vi "UTILITY Array Get 1D Column From 2D.vi"(0 "2D Array Data":dbl[][](array[numeric])=[[4000.0, 0.760276], [4100.0, 0.729117], [4200.0, 0.722886], [4300.0, 0.729117], [4400.0, 0.735349], [4500.0, 0.735349], [4600.0, 0.735349], [4700.0, 0.835058], [4800.0, 0.841289], [4900.0, 0.928534], [5000.0, 0.947229], [5100.0, 1.015779], [5200.0, 1.065633], [5300.0, 1.140414], [5400.0, 1.333599], [5500.0, 1.302441], [5600.0, 1.452003], [5700.0, 1.470698], [5800.0, 1.614029], [5900.0, 1.719969], [6000.0, 1.813446], [6100.0, 2.025326], [6200.0, 2.044021], [6300.0, 2.255902], [6400.0, 2.330683], [6500.0, 2.467782], [6600.0, 2.710821], [6700.0, 2.748212], [6800.0, 2.978787], [6900.0, 2.972556], [7000.0, 3.165741], [7100.0, 3.240522], [7200.0, 3.402548], [7300.0, 3.396316], [7400.0, 3.502256], [7500.0, 3.714137], [7600.0, 3.670514], [7700.0, 3.863699], [7800.0, 3.845004], [7900.0, 4.013262], [8000.0, 4.038189], [8100.0, 4.137897], [8200.0, 4.262533], [8300.0, 4.243837], [8400.0, 4.312387], [8500.0, 4.312387], [8600.0, 4.3934], [8700.0, 4.443254], [8800.0, 4.418327], [8900.0, 4.505572], [9000.0, 4.518035], [9100.0, 4.586585], [9200.0, 4.586585], [9300.0, 4.667598], [9400.0, 4.723684], [9500.0, 4.748611], [9600.0, 4.798465], [9700.0, 4.804697], [9800.0, 4.860783], [9900.0, 4.848319], [10000.0, 4.910637], [10100.0, 4.910637], [10200.0, 4.910637], [10300.0, 4.935564], [10400.0, 4.954259], [10500.0, 5.004114], [10600.0, 5.004114], [10700.0, 4.972955], [10800.0, 5.016577], [10900.0, 5.0602], [11000.0, 5.116285], [11100.0, 5.103822], [11200.0, 5.110054], [11300.0, 5.141213], [11400.0, 5.172371], [11500.0, 5.184835], [11600.0, 5.197299], [11700.0, 5.209762], [11800.0, 5.20353], [11900.0, 5.234689], [12000.0, 5.228457], [12100.0, 5.209762], [12200.0, 5.16614], [12300.0, 5.178603], [12400.0, 5.290775], [12500.0, 5.290775], [12600.0, 5.247153], [12700.0, 5.240921], [12800.0, 5.265848], [12900.0, 5.253384], [13000.0, 5.240921], [13100.0, 5.27208], [13200.0, 5.321934], [13300.0, 5.303239], [13400.0, 5.321934], [13500.0, 5.321934], [13600.0, 5.315702], [13700.0, 5.321934], [13800.0, 5.30947], [13900.0, 5.303239], [14000.0, 5.346861], [14100.0, 5.321934], [14200.0, 5.290775], [14300.0, 5.334398], [14400.0, 5.353093], [14500.0, 5.265848], [14600.0, 5.265848], [14700.0, 5.396715], [14800.0, 5.346861], [14900.0, 5.390483], [15000.0, 5.290775], [15100.0, 5.396715], [15200.0, 5.27208], [15300.0, 5.066431], [15400.0, 5.664682], [15500.0, 5.402947], [15600.0, 5.471497], [15700.0, 5.278312], [15800.0, 5.303239], [15900.0, 5.384252], [16000.0, 5.340629], [16100.0, 5.359325], [16200.0, 5.427874], [16300.0, 5.390483], [16400.0, 5.284543], [16500.0, 5.415411], [16600.0, 5.184835], [16700.0, 5.558741], [16800.0, 4.804697], [16900.0, 5.452801], [17000.0, 5.627291], [17100.0, 5.602364], [17200.0, 5.459033], [17300.0, 5.346861], [17400.0, 5.359325], [17500.0, 5.384252], [17600.0, 5.446569], [17700.0, 5.465265], [17800.0, 5.508887], [17900.0, 5.427874], [18000.0, 5.321934], [18100.0, 5.402947], [18200.0, 5.409179], [18300.0, 5.402947], [18400.0, 5.421642], [18500.0, 5.446569], [18600.0, 5.353093], [18700.0, 5.421642], [18800.0, 5.577437], [18900.0, 5.558741], [19000.0, 5.384252], [19100.0, 5.346861], [19200.0, 5.434106], [19300.0, 5.521351], [19400.0, 5.452801], [19500.0, 5.321934], [19600.0, 5.471497], [19700.0, 5.527583], [19800.0, 5.353093], [19900.0, 5.353093], [20000.0, 5.396715]] format="%0.3f", 7 "column index":i32) -> (4 "Column Data":dbl[](array[numeric]))   [LabVIEW 2020]
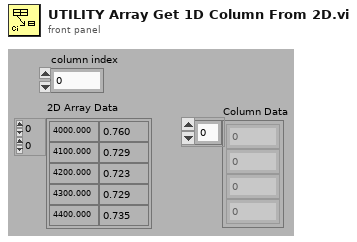
[diagram p1: front panel]
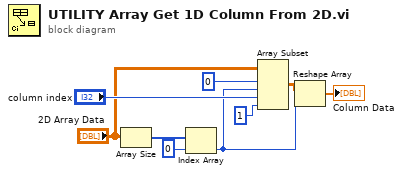
[diagram p0: block diagram]
diagram:
  n1 = Array Size(array="2D Array Data") -> (size(s)=w3:i32[])
  n2 = Index Array(array=w3, index=0) -> (element=w1:i32)
  n3 = Array Subset(array="2D Array Data", index (row)=0 ("index"), length (row)=w1, index (col)="column index", length (col)=1 ("length")) -> (w6:dbl[][])
  n4 = Reshape Array(w6, w1) -> (→"Column Data":dbl[])
